vi "Intake Loop.vi"   [LabVIEW 2015]
uses:
  Common Code/Intake States.ctl
  Robot Global Data.vi
types:
  T1 = typedef "Intake Commands Cluster.ctl" = cluster{"Intake Commands":T2, "Intake Mode":T3, "Override IR":bool}
  T2 = typedef "Intake Commands.ctl" = enum16{"Unload", "Load", "Pull up", "Drop low", "Idle", "Lift Half"}
  T3 = typedef "Intake Mode.ctl" = enum16{"Safe", "Auto", "Manual"}
  T4 = typedef "Dashboard Control Data.ctl" = cluster{"Shooter Presets":T5, "Encoder Control":T7, "Steer PID output":cluster{"output high":dbl, "output low":dbl}, " Steer PID gains":cluster{"proportional gain (Kc)":dbl, "integral time (Ti, min)":dbl, "derivative time (Td, min)":dbl}, "Drivetrain Settings":T8, "Vision Packet":T9, "Dashboard Drivetrain Command":T10, "Info/Command Cluster":T12, "Ball Vision Packet":T13, "Intake Presets":T15, "Intake Encoder Control":T17, "Climb Presets":T18, "Ultrasonic Limit":dbl, "Roll Limit":dbl, "Pitch Limit":dbl, "Goal Output Range":cluster{"output high":dbl, "output low":dbl}}
  T5 = typedef "Shooter Presets.ctl" = cluster{"Batter Shot":T6, "Deep Middle Shot":T6, "Manual Shot":T6, "Left Ticks Per Rotation":dbl, "Right Ticks Per Rotation":dbl, "Low Bar Shot":T6, "Shooter RPM Tolerance":dbl, "IIR Filter Power":dbl, "Trigger Power":dbl, "Fire from Load Delay":i32, "Angle Pot M":dbl, "Angle Pot B":dbl, "Shooter Length":dbl, "String Pot Dist":dbl, "Angle PID gains":cluster{"proportional gain (Kc)":dbl, "integral time (Ti, min)":dbl, "derivative time (Td, min)":dbl}, "Angle Motor Output":cluster{"output high":dbl, "output low":dbl}, "Shooter Angle Tolerance":dbl, "Vision Shoot x^2":dbl, "Vision Shoot x":dbl, "Dist from Axis Cam to Pivot":dbl, "High Goal Center Height":dbl, "Feed Forward Max Accel":dbl, "Feed Forward Kv":dbl, "Backwards Trigger":dbl, "Shot Finish Delay (ms)":dbl, "Angle Max Current":dbl, "Angle Current Trip Time":dbl, "Shooter Intake Angle":dbl, "Vision Shoot c":dbl, "Reset?":bool, "Servo Release Delay":dbl, "Servo Idle Angle":i32, "Servo Hold Angle":i32, "Angle Pot x^2":dbl, "Angle Pot x":dbl, "Angle Pot c":dbl, "Ignore Angle?":bool}
  T6 = typedef "Shot Presets.ctl" = cluster{"Left Wheel RPM":dbl, "Right Wheel RPM":dbl, "Angle":dbl}
  T7 = typedef "Encoder Control.ctl" = cluster{"Right Tick Constant":dbl, "Left Tick Constant":dbl, "Reset?":bool, "Y Dist":cluster{"PID gains":cluster{"proportional gain (Kc)":dbl, "integral time (Ti, min)":dbl, "derivative time (Td, min)":dbl}}, "Y Stop Thresh":dbl, "Y Stop Speed":dbl}
  T8 = typedef "Drivetrain Settings.ctl" = cluster{"Gyro Tolerance":dbl, "Throttle Ramp (ms)":dbl, "Angular rate compensation":bool, "Throttle to Rate Scale":dbl, "Rate compensation gain":dbl, "Kv":dbl, "Ka":dbl, "Feed Forward P":dbl, "Feed Forward D":dbl, "Goal Vision PID gains":cluster{"proportional gain (Kc)":dbl, "integral time (Ti, min)":dbl, "derivative time (Td, min)":dbl}, "Goal Detection Window":dbl}
  T9 = typedef "Goal Vision Packet.ctl" = cluster{"Distance":dbl, "Center X":dbl, "Center Y":dbl, "Found Target?":bool}
  T10 = typedef "Dashboard Drivetrain Command.ctl" = cluster{"Drivetrain Vision":T11}
  T11 = typedef "Drivetrain Vision.ctl" = cluster{"Goal Window":dbl, "Ball Window":dbl}
  T12 = typedef "Ball Tracking Command Cluster.ctl" = cluster{"Distance to Ball":dbl, "Desired Angle":dbl, "Command":enum16{"Turn to Ball", "Turn to Angle", "Get Distance"}, "Pixels from Center":dbl}
  T13 = typedef "Ball Vision Packet.ctl" = cluster{"Ball Detected?":bool, "Distance to Ball":dbl, "Desired Angle":dbl, "Pixels from Center":dbl, "Tracking mode":T14}
  T14 = typedef "Tracking Mode.ctl" = enum16{"Turn to Ball", "Turn to Angle"}
  T15 = typedef "Intake Presets.ctl" = cluster{"Intake Speed":dbl, "Outake Speed":dbl, "Low Height":dbl, "Half Height":dbl, "Full Height":dbl, "Angle Speed":dbl, "Fast Angle":dbl, "Encoder Scale":dbl, "Load Height":dbl, "Output Range":T16, "Rotation Power Max/Min":dbl, "MaxCurrent":dbl, "Intake Trip Time":dbl, "Idle Height":dbl, "Max Height":dbl, "Reset Encoders?":bool, "PID gains":cluster{"proportional gain (Kc)":dbl, "integral time (Ti, min)":dbl, "derivative time (Td, min)":dbl}}
  T16 = typedef "Drivetrain Output Range.ctl" = cluster{"output high":dbl, "output low":dbl}
  T17 = typedef "IntakeEcoderControl.ctl" = cluster{"Arm Tick Constant":dbl, "Reset?":bool, "Y Dist":cluster{"PID gains":cluster{"proportional gain (Kc)":dbl, "integral time (Ti, min)":dbl, "derivative time (Td, min)":dbl}}, "Y Stop Thresh":dbl, "Y Stop Speed":dbl}
  T18 = typedef "Climb Presets.ctl" = cluster{"Pull Power":dbl, "Unpin Power":dbl, "Time to Hold":dbl}
  T19 = typedef "WPI_MotorControlDeviceRef.ctl" = cluster{"DeviceStatus":errorcluster, "Type":T20, "PWM":cluster{"PWM Channel":T21, "DeadBand":T22}, "CAN":cluster{"Device Number":u8, "Control Mode":T23, "Semaphore":T24, "Max Vout":dbl, "TalonSRX Control Mode":T25}, "Invert":bool}
  T20 = typedef "WPI_MotorControlType.ctl" = enum16{"PWM", "CAN", "CANTalonSRX"}
  T21 = typedef "FPGA_DIOPWMChannel.ctl" = enum8{"PWM 0", "PWM 1", "PWM 2", "PWM 3", "PWM 4", "PWM 5", "PWM 6", "PWM 7", "PWM 8", "PWM 9", "PWM MXP 0", "PWM MXP 1", "PWM MXP 2", "PWM MXP 3", "PWM MXP 4", "PWM MXP 5", "PWM MXP 6", "PWM MXP 7", "PWM MXP 8", "PWM MXP 9", "Invalid"}
  T22 = typedef "WPI_PWMDeadband.ctl" = cluster{"Name":string, "maxPositivePwm":i32, "minPositivePwm":i32, "centerPwm":i32, "maxNegativePwm":i32, "minNegativePwm":i32, "angularRange":u16}
  T23 = typedef "WPI_CANJaguar_ControlMode.ctl" = enum8{"Percent VBus", "Current", "Speed", "Position", "Voltage"}
  T24 = typedef "Semaphore RefNum" = refnum<k1>
  T25 = typedef "WPI_CANTalonSRX_APIControlMode.ctl" = enum8{"Percent VBus", "Speed", "Position", "Slave", "Unchanged / Invalid", "Voltage Compensation", "Current", "Motion Profile"}
  T26 = typedef "Intake States.ctl" = enum16{"Idle", "Set roller speed", "Move to angle"}
  T27 = typedef "Intake Status Cluster.ctl" = cluster{"Roller Power":dbl, "Angle Power":dbl, "Intake Mode":T3, "Intake States":T26, "Rollers Active?":bool, "Current Height":dbl, "Target Height":dbl, "Encoder Raw Position":dbl, "Forward Tripped?":bool, "Backward Tripped?":bool, "Override IR?":bool}
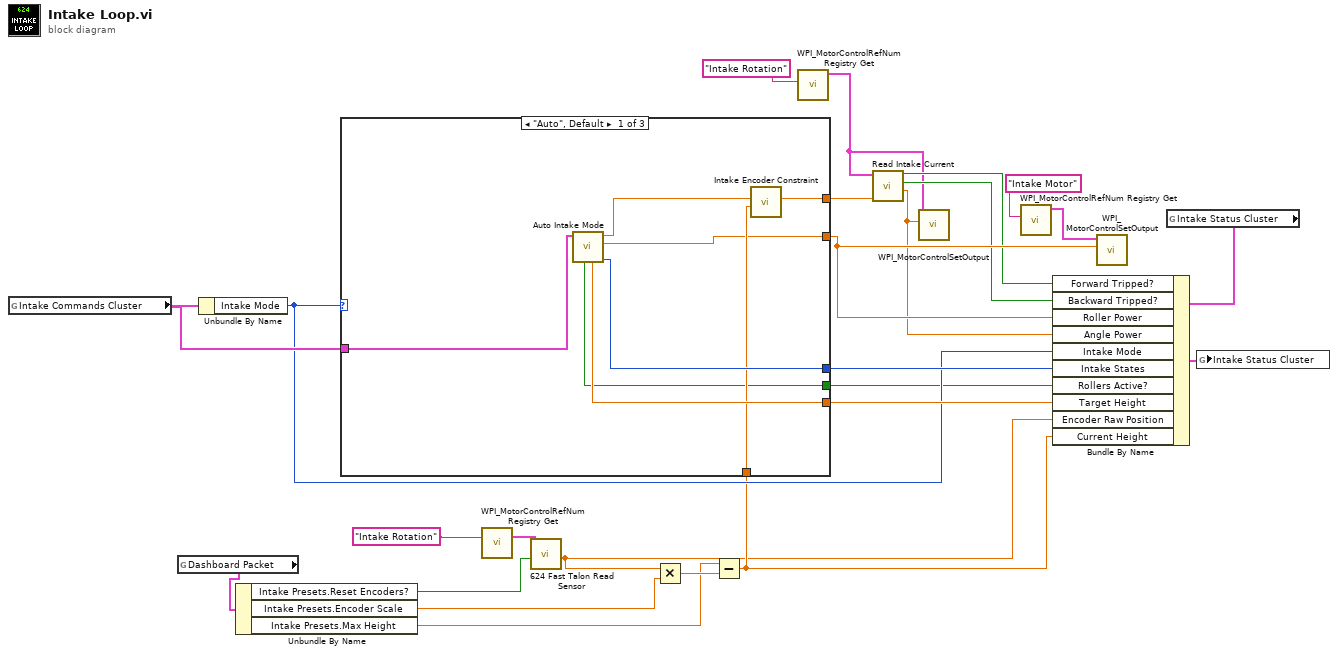
[diagram p0: block diagram]
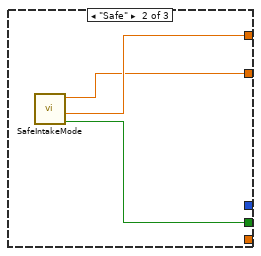
[diagram p2: hidden frame]
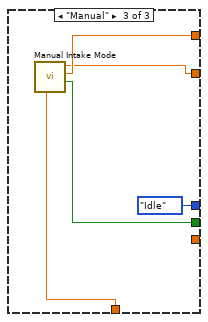
[diagram p3: hidden frame]
diagram:
  n1 = global read "Robot Global Data.vi" "Intake Commands Cluster"() -> (w25:T1)
  n2 = global read "Robot Global Data.vi" "Dashboard Packet"() -> (w4:T4)
  n3 = Unbundle By Name(w25) -> ("Intake Mode"=w17:T3)
  n4 = Unbundle By Name(w4) -> ("Intake Presets.Reset Encoders?"=w2:bool, "Intake Presets.Encoder Scale"=w6:dbl, "Intake Presets.Max Height"=w5:dbl)
  n5 = call <vilib>:"WPI_MotorControlRefNum Registry Get.vi"("refnum name"="Intake Rotation") -> ("MotorControlDevRef"=w14:T19)  [unwired: 9 in, 1 out]
  n6 = call "624 Fast Talon Read Sensor.vi"("Reset?"=w2, "MotorControlDevRef"=w14) -> ("Current"=w3:dbl)  [unwired: 6 in, 3 out]
  n7 = Multiply(x=w3, y=w6) -> (x*y=w7:dbl)
  n8 = Subtract(x=w5, y=w7) -> (x-y=w8:dbl)
  n9 = case shown="\"Auto\", Default" w17 {
    tunnel: w25 -> [w33 _ _]
    tunnel: [w26 w36 w40] -> w13
    tunnel: [w27 w35 w39] -> w21
    tunnel: [w31 _ Intake_States."Idle" ("Intake States")] -> w19
    tunnel: [w32 _ _] -> w18
    tunnel: w8 -> [w30 _ w37]
    tunnel: [w29 w34 w38] -> w9
    frame "Auto", Default {
      n10 = call "Auto Intake Mode.vi"("Intake Commands Cluster"=w33) -> ("Intake States"=w31:T26, "Roller Power"=w27:dbl, "Angle Power"=w28:dbl, "Target Height"=w32:dbl, "Rollers Active?"=w29:bool)  [unwired: 4 in, 2 out]
      n11 = call "Intake Encoder Constraint.vi"("Arm Power"=w28, "Encoder Position"=w30) -> ("Roller Power"=w26:dbl)  [unwired: 8 in]
    }
    frame "Safe" {
      n12 = call "SafeIntakeMode.vi"() -> ("Rollers Active?"=w34:bool, "Angle Power"=w36:dbl, "Roller Power"=w35:dbl)  [unwired: 9 in]
    }
    frame "Manual" {
      n13 = call "Manual Intake Mode.vi"("Current Encoder Position"=w37) -> ("Rollers Active?"=w38:bool, "Arm Power"=w40:dbl, "Intake Power"=w39:dbl)  [unwired: 8 in]
    }
  }
  n14 = call <vilib>:"WPI_MotorControlRefNum Registry Get.vi"("refnum name"="Intake Rotation") -> ("MotorControlDevRef"=w1:T19)  [unwired: 9 in, 1 out]
  n15 = call "Read Intake Current.vi"("Proposed Power"=w13, "CAN Talon SRX Ref"=w1) -> ("Actual Power"=w12:dbl, "Reverse Trip?"=w10:bool, "Forward Trip?"=w11:bool)  [unwired: 7 in]
  n16 = call <vilib>:"WPI_MotorControlSetOutput.vi"("Output"=w12, "MotorControlDevRef"=w1) -> ()  [unwired: 7 in, 3 out]
  n17 = call <vilib>:"WPI_MotorControlRefNum Registry Get.vi"("refnum name"="Intake Motor") -> ("MotorControlDevRef"=w23:T19)  [unwired: 9 in, 1 out]
  n18 = call <vilib>:"WPI_MotorControlSetOutput.vi"("Output"=w21, "MotorControlDevRef"=w23) -> ()  [unwired: 7 in, 3 out]
  n19 = global read "Robot Global Data.vi" "Intake Status Cluster"() -> (w16:T27)
  n20 = Bundle By Name(cluster=w16, "Forward Tripped?"=w11, "Backward Tripped?"=w10, "Roller Power"=w21, "Angle Power"=w12, "Intake Mode"=w17, "Intake States"=w19, "Rollers Active?"=w9, "Target Height"=w18, "Encoder Raw Position"=w3, "Current Height"=w8) -> (w20:T27)
  n21 = global write "Robot Global Data.vi" "Intake Status Cluster"(w20) -> ()
